vi "Format Technique.vi"(8 "error in (no error)":errorcluster, 9 "Technique in":T1, 10 "Technique Parameters in":variant, 11 "Potentiostat Galvanostat in":refnum<class "Potentiostat Galvanostat.lvclass">) -> (0 "error out":errorcluster, 1 "Technique Parameters out":T2 {"Parameter Type" items=["I32 (Long)", "BOOL (Boolean)", "SGL (Single Precision)"]}, 3 "Potentiostat Galvanostat out":refnum<class "Potentiostat Galvanostat.lvclass">)   [LabVIEW 2018, in "Potentiostat Galvanostat.lvclass"]
uses:
  Potentiostat Galvanostat.lvclass
  Controls/Technique Parameters.ctl
  Controls/Technique Parameter.ctl
  Controls/Parameter Type.ctl
  Controls/Technique List.ctl
  Controls/Error Codes.ctl
  Controls/OCV Parameters.ctl
  Controls/CV Parameters.ctl
  Controls/CA Parameters.ctl
  Controls/CP Parameters.ctl
  Controls/PEIS Parameters.ctl
  Controls/GEIS Parameters.ctl
  <vilib>/Utility/Data Type/NI_Data Type.lvlib
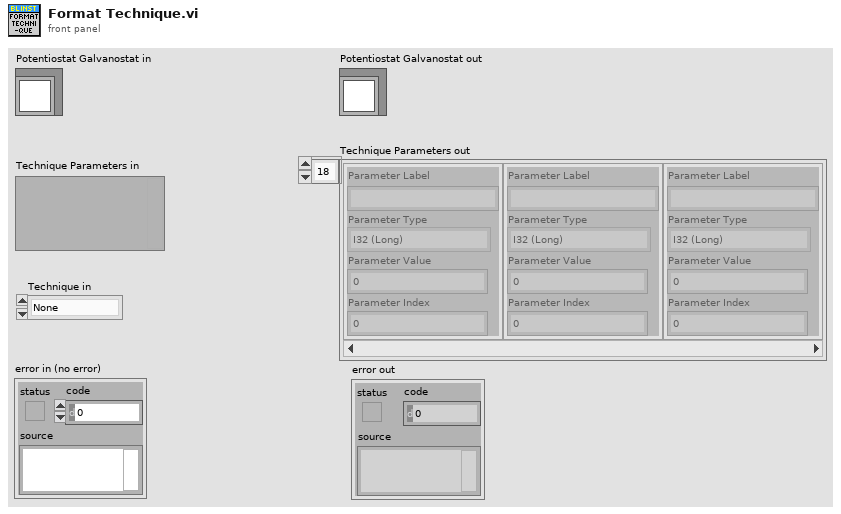
[diagram p1: front panel]
types:
  T1 = typedef "Potentiostat Galvanostat.lvclass/Technique List.ctl" = enum16{"None", "ocv", "cv", "biovscan", "ca", "cp", "iscan", "vscan", "lasv", "load", "pow", "peis", "geis", "seisp", "seisg", "dpv", "swv", "npv", "mpv", "dnpv", "dpa", "evt", "lp", "gc", "cpp", "pdp", "psp", "zra", "ircmp", "pzir", "gzir", "loop", "TO", "TI", "TOS", "vscanlimit", "iscanlimit", "mp", "casp", "casg", "calimit", "cplimit"}
  T2 = typedef "Potentiostat Galvanostat.lvclass/Technique Parameters.ctl" = T3[]
  T3 = typedef "Potentiostat Galvanostat.lvclass/Technique Parameter.ctl" = cluster{"Parameter Label":string, "Parameter Type":T4, "Parameter Value":i32, "Parameter Index":i32}
  T4 = typedef "Potentiostat Galvanostat.lvclass/Parameter Type.ctl" = i32
  T5 = typedef "Potentiostat Galvanostat.lvclass/OCV Parameters.ctl" = cluster{"Rest_time_T":sgl, "Record_every_dE":sgl, "Record_every_dT":sgl, "E_Range":u16, "em":u16, "ce":u16, "tb":sgl}
  T6 = typedef "Potentiostat Galvanostat.lvclass/CV Parameters.ctl" = cluster{"Ei Params":cluster{"vs_initial":bool, "Voltage_step":sgl, "Scan_Rate":sgl}, "E1 Params":cluster{"vs_initial":bool, "Voltage_step":sgl, "Scan_Rate":sgl}, "E2 Params":cluster{"vs_initial":bool, "Voltage_step":sgl, "Scan_Rate":sgl}, "Ef Params":cluster{"vs_initial":bool, "Voltage_step":sgl, "Scan_Rate":sgl}, "N_Cycles":i32, "Record_every_dE":sgl, "Average_over_dE":bool, "Begin_measuring_I":sgl, "End_measuring_I":sgl, "I_Range":u16, "E_Range":u16, "Bandwidth":u16, "em":u16, "ce":u16, "Scan_number":u16}
  T7 = typedef "Potentiostat Galvanostat.lvclass/CA Parameters.ctl" = cluster{"tb":sgl, "Steps":cluster{"vs_initial":bool, "Voltage_step":sgl, "Duration_step":sgl}[], "Step_number":i32, "N_Cycles":i32, "Record_every_dI":sgl, "Record_every_dT":sgl, "I_Range":u16, "E_Range":u16, "Bandwidth":u16, "em":u16, "ce":u16}
  T8 = typedef "Potentiostat Galvanostat.lvclass/CP Parameters.ctl" = cluster{"Steps":cluster{"vs_initial":bool, "Current_step":sgl, "Duration_step":sgl}[], "Step_number":i32, "N_Cycles":i32, "Record_every_dE":sgl, "Record_every_dT":sgl, "I_Range":u16, "E_Range":u16, "Bandwidth":u16, "em":u16, "ce":u16, "tb":sgl}
  T9 = typedef "Potentiostat Galvanostat.lvclass/PEIS Parameters.ctl" = cluster{"Step_number":i32, "Initial_Voltage_step":sgl, "vs_initial":bool, "Final_Voltage_step":sgl, "vs_final":bool, "Duration_step":sgl, "Record_every_dI":sgl, "Record_every_dT":sgl, "Initial_frequency":sgl, "sweep":bool, "Final_frequency":sgl, "Frequency_number":i32, "Amplitude_Voltage":sgl, "Wait_for_steady":sgl, "Average_N_times":i32, "Correction":bool, "I_Range":u16, "Bandwidth":u16, "em":u16, "ce":u16}
  T10 = typedef "Potentiostat Galvanostat.lvclass/GEIS Parameters.ctl" = cluster{"Step_number":i32, "Initial_Current_step":sgl, "vs_initial ":bool, "Final_Current_step":sgl, "vs_final":bool, "Duration_step":sgl, "Record_every_dE":sgl, "Record_every_dT":sgl, "Initial_frequency":sgl, "sweep":bool, "Final_frequency":sgl, "Frequency_number":i32, "Amplitude_Current":sgl, "Wait_for_steady":sgl, "Average_N_times":i32, "Correction":bool, "I_Range":u16, "Bandwidth":u16, "em":u16, "ce":u16}
  T11 = typedef "Potentiostat Galvanostat.lvclass/Error Codes.ctl" = i32
  T12 = cluster{"vs_initial":bool, "Voltage_step":sgl, "Scan_Rate":sgl}
  T13 = cluster{"vs_initial":bool, "Voltage_step":sgl, "Scan_Rate":sgl}[]
  T14 = typedef "NI_Data Type.lvlib/Data Type.ctl" = enum8{"Invalid Type", "Void", "I8", "I16", "I32", "I64", "U8", "U16", "U32", "U64", "Single Float", "Double Float", "Extended Float", "Single Complex", "Double Complex", "Extended Complex", "Enum U8", "Enum U16", "Enum U32", "Enum U64", "Single Float With Unit", "Double Float With Unit", "Extended Float With Unit", "Single Complex with Unit", "Double Complex with Unit", "Extended Complex with Unit", "Boolean", "String", "Path", "Picture", "Tag", "Array", "Cluster", "Variant", "LV Variant", "Waveform", "Timestamp", "Digital Waveform", "Digital Data", "ExpressData", "Refnum", "External Data", "VI", "Poly VI", "LabVIEW Class Instance", "Fixed Point"}
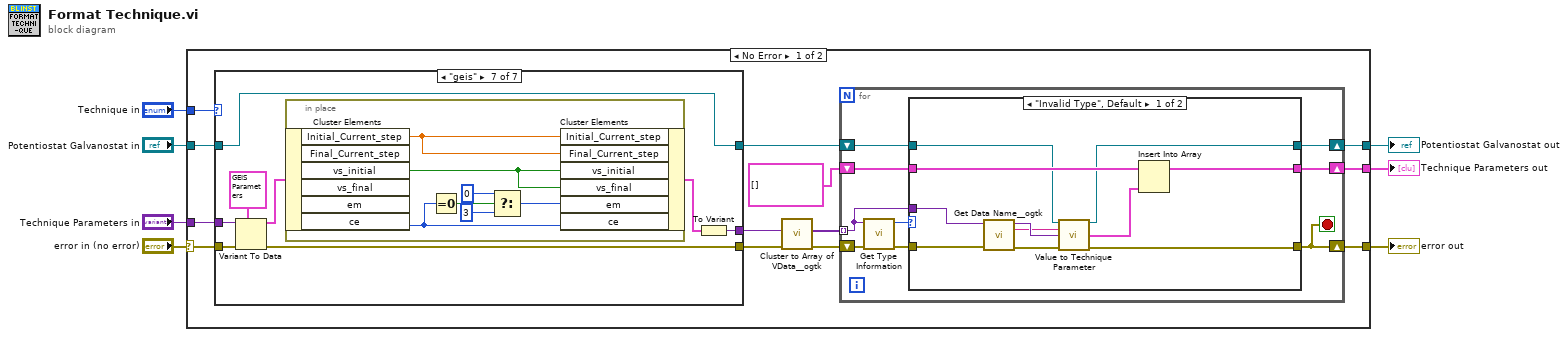
[diagram p0: block diagram]
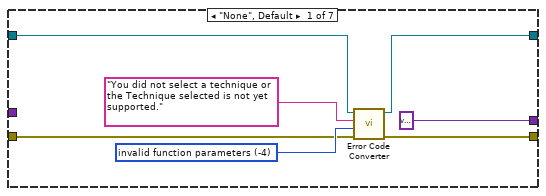
[diagram p2: hidden frame]
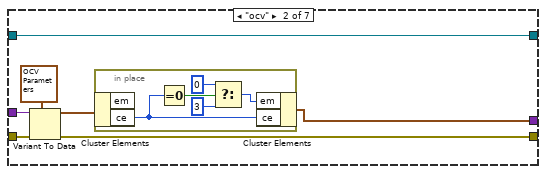
[diagram p3: hidden frame]
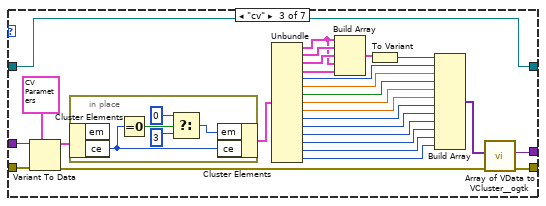
[diagram p4: hidden frame]
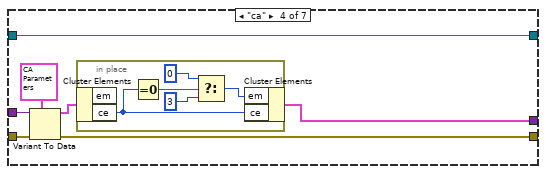
[diagram p5: hidden frame]
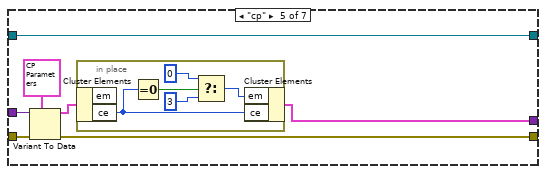
[diagram p6: hidden frame]
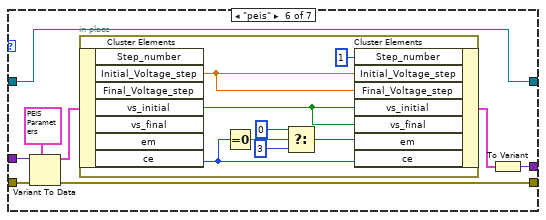
[diagram p7: hidden frame]
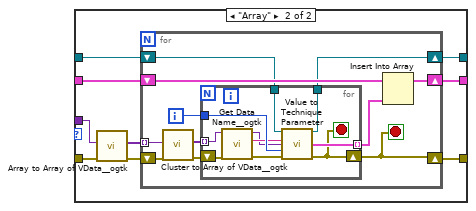
[diagram p8: hidden frame]
diagram:
  n1 = case shown="No Error" "error in (no error)" {
    selector: "error in (no error)" -> [w14 w178]
    tunnel: "Technique Parameters in" -> [w13 _]
    tunnel: "Potentiostat Galvanostat in" -> [w12 w177]
    tunnel: [w11 w178] -> w2
    tunnel: [w10 w177] -> w4
    tunnel: [w9 _] -> w3
    tunnel: "Technique in" -> [w8 _]
    frame No Error {
      n2 = case shown="\"geis\"" w8 {
        tunnel: w13 -> [_ w34 w66 w78 w90 w102 w119]
        tunnel: [w26 w30 w45 w72 w86 w98 w115] -> w17
        tunnel: w14 -> [w25 w33 w65 w76 w88 w100 w117]
        tunnel: [w22 w29 w64 w73 w85 w96 w113] -> w15
        tunnel: w12 -> [w23 w29 w64 w73 w85 w96 w113]
        tunnel: [variant ("Variant") w28 w44 w74 w84 w97 w114] -> w16
        frame "None", Default {
          w27 = T11 -4 items=["No Error"=0, "no instrument connected"=-1, "connection in progress"=-2, "selected channel(s) unplugged"=-3, "invalid function parameters"=-4, "selected file does not exist"=-5, "function failed"=-6, "no channel selected"=-7, "invalid instrument configuration"=-8, "EC-Lab firmware loaded on the instrument"=-9, "library not correctly loaded in memory"=-10, "USB library not correctly loaded in memory"=-11, "function of the library already in progress"=-12, "selected channel(s) already used"=-13, "device not allowed"=-14, "Invalid update function parameters"=-15, "internal instrument communication failed"=-101, "too many data to transfer from the instrument (device error)"=-102, "selected channel(s) unplugged (device error)"=-103, "instrument response error"=-104, "invalid message size"=-105] ("Error Code")
          n3 = call-dynamic "Error Code Converter.vi"("error in (no error)"=w25, "Error Code"=w27, "Additional Description"="You did not select a technique or the Technique selected is not yet supported.", "Potentiostat Galvanostat in"=w23) -> ("error out"=w26:errorcluster, "Potentiostat Galvanostat out"=w22:refnum<class "Potentiostat Galvanostat.lvclass">)  [unwired: 6 in]
        }
        frame "ocv" {
          n4 = Variant To Data(error in=w33, type=T5 {"Rest_time_T"=1.0, "Record_every_dE"=0.01, "Record_every_dT"=0.01, "E_Range"=3, "em"=1, "ce"=0, "tb"=2e-05} ("OCV Parameters"), Variant=w34) -> (data=w32:T5, error out=w30:errorcluster)
          n5 = in-place {
            n6 = in-place-cluster #1(w32) -> ("ce"=w35:u16)  [unwired: 1 out]
            n7 = Equal To 0?(x=w35) -> (x = 0?=w39:bool)
            n8 = Select(t=u16 0, s=w39, f=u16 3) -> (s? t:f=w36:u16)
            n9 = in-place-cluster #1("em"=w36, "ce"=w35) -> (w28:T5)
          }
        }
        frame "cv" {
          n10 = Variant To Data(error in=w65, type=T6 {"Ei Params"={"vs_initial"=FALSE, "Voltage_step"=0.0, "Scan_Rate"=0.1}, "E1 Params"={"vs_initial"=FALSE, "Voltage_step"=0.1, "Scan_Rate"=0.1}, "E2 Params"={"vs_initial"=FALSE, "Voltage_step"=-0.2, "Scan_Rate"=0.1}, "Ef Params"={"vs_initial"=FALSE, "Voltage_step"=0.0, "Scan_Rate"=0.1}, "N_Cycles"=1, "Record_every_dE"=0.01, "Average_over_dE"=TRUE, "Begin_measuring_I"=0.5, "End_measuring_I"=0.75, "I_Range"=12, "E_Range"=3, "Bandwidth"=5, "em"=1, "ce"=0, "Scan_number"=2} ("CV Parameters"), Variant=w66) -> (data=w63:T6, error out=w43:errorcluster)
          n11 = in-place {
            n12 = in-place-cluster #2(w63) -> ("ce"=w68:u16)  [unwired: 1 out]
            n13 = Equal To 0?(x=w68) -> (x = 0?=w71:bool)
            n14 = Select(t=u16 0, s=w71, f=u16 3) -> (s? t:f=w69:u16)
            n15 = in-place-cluster #2("em"=w69, "ce"=w68) -> (w41:T6)
          }
          n16 = Unbundle(w41) -> ("Ei Params"=w59:T12, "E1 Params"=w62:T12, "E2 Params"=w61:T12, "Ef Params"=w60:T12, "N_Cycles"=w56:i32, "Record_every_dE"=w55:sgl, "Average_over_dE"=w54:bool, "Begin_measuring_I"=w53:sgl, "End_measuring_I"=w52:sgl, "I_Range"=w51:u16, "E_Range"=w50:u16, "Bandwidth"=w49:u16, "em"=w48:u16, "ce"=w47:u16, "Scan_number"=w46:u16)
          n17 = Build Array(w59, w62, w61, w59, w60) -> (w58:T13)
          n18 = To Variant(anything=w58) -> (Variant=w57:variant)
          n19 = Build Array(w57, w56, w55, w54, w53, w52, w51, w50, w49, w48, w47, w46) -> (w42:variant[])
          n20 = call <userlib>:"Array of VData to VCluster__ogtk.vi"("error in (no error)"=w43, "Array"=w42) -> ("error out"=w45:errorcluster, "VCluster"=w44:variant)  [unwired: 8 in]
        }
        frame "ca" {
          n21 = Variant To Data(error in=w76, type=T7 {"tb"=2.5e-05, "Steps"=[{"vs_initial"=TRUE, "Voltage_step"=0.0, "Duration_step"=1.0}, {"vs_initial"=TRUE, "Voltage_step"=0.1, "Duration_step"=1.0}, {"vs_initial"=TRUE, "Voltage_step"=0.2, "Duration_step"=1.0}], "Step_number"=2, "N_Cycles"=0, "Record_every_dI"=1e-05, "Record_every_dT"=0.01, "I_Range"=8, "E_Range"=3, "Bandwidth"=5, "em"=1, "ce"=0} ("CA Parameters"), Variant=w78) -> (data=w77:T7, error out=w72:errorcluster)
          n22 = in-place {
            n23 = in-place-cluster #3(w77) -> ("ce"=w79:u16)  [unwired: 1 out]
            n24 = Equal To 0?(x=w79) -> (x = 0?=w83:bool)
            n25 = Select(t=u16 0, s=w83, f=u16 3) -> (s? t:f=w80:u16)
            n26 = in-place-cluster #3("em"=w80, "ce"=w79) -> (w74:T7)
          }
        }
        frame "cp" {
          n27 = Variant To Data(error in=w88, type=T8 {"Steps"=[{"vs_initial"=FALSE, "Current_step"=0.0, "Duration_step"=1.0}, {"vs_initial"=FALSE, "Current_step"=0.001, "Duration_step"=1.0}, {"vs_initial"=FALSE, "Current_step"=0.005, "Duration_step"=1.0}], "Step_number"=2, "N_Cycles"=0, "Record_every_dE"=0.005, "Record_every_dT"=0.05, "I_Range"=8, "E_Range"=3, "Bandwidth"=5, "em"=1, "ce"=0, "tb"=2.5e-05} ("CP Parameters"), Variant=w90) -> (data=w89:T8, error out=w86:errorcluster)
          n28 = in-place {
            n29 = in-place-cluster #4(w89) -> ("ce"=w91:u16)  [unwired: 1 out]
            n30 = Equal To 0?(x=w91) -> (x = 0?=w95:bool)
            n31 = Select(t=u16 0, s=w95, f=u16 3) -> (s? t:f=w92:u16)
            n32 = in-place-cluster #4("em"=w92, "ce"=w91) -> (w84:T8)
          }
        }
        frame "peis" {
          n33 = Variant To Data(error in=w100, type=T9 {"Step_number"=0, "Initial_Voltage_step"=0.0, "vs_initial"=TRUE, "Final_Voltage_step"=1.0, "vs_final"=FALSE, "Duration_step"=1.0, "Record_every_dI"=0.1, "Record_every_dT"=0.1, "Initial_frequency"=100000.0, "sweep"=FALSE, "Final_frequency"=1.0, "Frequency_number"=51, "Amplitude_Voltage"=0.01, "Wait_for_steady"=2.0, "Average_N_times"=1, "Correction"=TRUE, "I_Range"=12, "Bandwidth"=5, "em"=1, "ce"=0} ("PEIS Parameters"), Variant=w102) -> (data=w101:T9, error out=w98:errorcluster)
          n34 = in-place {
            n35 = in-place-cluster #5(w101) -> ("Initial_Voltage_step"=w111:sgl, "vs_initial"=w104:bool, "ce"=w106:u16)  [unwired: 4 out]
            n36 = Equal To 0?(x=w106) -> (x = 0?=w110:bool)
            n37 = Select(t=u16 0, s=w110, f=u16 3) -> (s? t:f=w107:u16)
            n38 = in-place-cluster #5("Step_number"=1, "Initial_Voltage_step"=w111, "Final_Voltage_step"=w111, "vs_initial"=w104, "vs_final"=w104, "em"=w107, "ce"=w106) -> (w99:T9)
          }
          n39 = To Variant(anything=w99) -> (Variant=w97:variant)
        }
        frame "geis" {
          n40 = Variant To Data(error in=w117, type=T10 {"Step_number"=0, "Initial_Current_step"=0.0, "vs_initial "=TRUE, "Final_Current_step"=0.001, "vs_final"=TRUE, "Duration_step"=1.0, "Record_every_dE"=0.1, "Record_every_dT"=0.1, "Initial_frequency"=100000.0, "sweep"=FALSE, "Final_frequency"=1.0, "Frequency_number"=51, "Amplitude_Current"=0.001, "Wait_for_steady"=2.0, "Average_N_times"=1, "Correction"=TRUE, "I_Range"=7, "Bandwidth"=5, "em"=1, "ce"=0} ("GEIS Parameters"), Variant=w119) -> (data=w118:T10, error out=w115:errorcluster)
          n41 = in-place {
            n42 = in-place-cluster #6(w118) -> ("Initial_Current_step"=w126:sgl, "vs_initial"=w120:bool, "ce"=w121:u16)  [unwired: 3 out]
            n43 = Equal To 0?(x=w121) -> (x = 0?=w125:bool)
            n44 = Select(t=u16 0, s=w125, f=u16 3) -> (s? t:f=w122:u16)
            n45 = in-place-cluster #6("Initial_Current_step"=w126, "Final_Current_step"=w126, "vs_initial"=w120, "vs_final"=w120, "em"=w122, "ce"=w121) -> (w116:T10)
          }
          n46 = To Variant(anything=w116) -> (Variant=w114:variant)
        }
      }
      n47 = call <userlib>:"Cluster to Array of VData__ogtk.vi"("error in (no error)"=w17, "Cluster"=w16) -> ("error out"=w20:errorcluster, "Array of VData"=w19:variant[])  [unwired: 8 in]
      n48 = for {
        tunnel: w19 -> [w132] mode=indexing
        shift-right: [w130] -> w9
        shift-left: T2 [] ("Technique Parameters") -> [w135]
        shift-right: [w127] -> w11
        shift-left: w20 -> [w134]
        shift-right: [w128] -> w10
        shift-left: w15 -> [w129]
        stop <- w127 stop-if-true
        n49 = call <vilib>:"Get Type Information.vi"("error in (no error)"=w134, "Variant"=w132) -> ("error out"=w131:errorcluster, "Type"=w133:T14)  [unwired: 5 in, 3 out]
        n50 = case shown="\"Invalid Type\", Default" w133 {
          tunnel: w132 -> [w142 w155]
          tunnel: [w138 w152] -> w130
          tunnel: w135 -> [w141 w151]
          tunnel: w131 -> [w146 w150]
          tunnel: [w139 w149] -> w127
          tunnel: w129 -> [w137 w148]
          tunnel: [w136 w147] -> w128
          frame "Invalid Type", Default {
            n51 = call <userlib>:"Get Data Name__ogtk.vi"("error in (no error)"=w146, "Data"=w142) -> ("error out"=w145:errorcluster, "Data Name"=w143:string, "Data dup"=w144:variant)  [unwired: 7 in]
            n52 = call-dynamic "Value to Technique Parameter.vi"("Potentiostat Galvanostat in"=w137, "Parameter Label"=w143, "Parameter Value"=w144, "error in (no error)"=w145) -> ("Potentiostat Galvanostat out"=w136:refnum<class "Potentiostat Galvanostat.lvclass">, "Technique Parameter"=w140:T3, "error out"=w139:errorcluster)  [unwired: 9 in]
            n53 = Insert Into Array(array=w141, new element=w140) -> (w138:T2)  [unwired: 1 in]
          }
          frame "Array" {
            n54 = call <userlib>:"Array to Array of VData__ogtk.vi"("error in (no error)"=w150, "MultiD Array"=w155) -> ("error out"=w153:errorcluster, "1D Array of Variants"=w154:variant[])  [unwired: 8 in]
            n55 = for {
              tunnel: w154 -> [w166] mode=indexing
              shift-right: [w159] -> w152
              shift-left: w151 -> [w161]
              shift-right: [w156] -> w149
              shift-left: w153 -> [w162]
              shift-right: [w157] -> w147
              shift-left: w148 -> [w158]
              i -> [w163]
              stop <- w156 stop-if-true
              n56 = call <userlib>:"Cluster to Array of VData__ogtk.vi"("error in (no error)"=w162, "Cluster"=w166) -> ("error out"=w164:errorcluster, "Array of VData"=w165:variant[])  [unwired: 8 in]
              n57 = for {
                tunnel: w165 -> [w172] mode=indexing
                tunnel: w163 -> [w174]
                tunnel: [w170] -> w160 mode=indexing
                shift-right: [w167] -> w156
                shift-left: w164 -> [w175]
                tunnel: w158 -> [w169]
                tunnel: [w168] -> w157
                stop <- w167 stop-if-true
                n58 = call <userlib>:"Get Data Name__ogtk.vi"("error in (no error)"=w175, "Data"=w172) -> ("error out"=w176:errorcluster, "Data Name"=w173:string, "Data dup"=w171:variant)  [unwired: 7 in]
                n59 = call-dynamic "Value to Technique Parameter.vi"("Potentiostat Galvanostat in"=w169, "Parameter Label"=w173, "Parameter Value"=w171, "Parameter Index"=w174, "error in (no error)"=w176) -> ("Potentiostat Galvanostat out"=w168:refnum<class "Potentiostat Galvanostat.lvclass">, "Technique Parameter"=w170:T3, "error out"=w167:errorcluster)  [unwired: 8 in]
              }
              n60 = Insert Into Array(array=w161, new element=w160) -> (w159:T2)  [unwired: 1 in]
            }
          }
        }
      }
    }
    frame Error {
    }
  }
  "error out" <- w2
  "Potentiostat Galvanostat out" <- w4
  "Technique Parameters out" <- w3
